vi "img test9(track 2_ num of particles).vi"() -> ()   [LabVIEW 2013]
uses:
  <vilib>/vision/NI_Vision_Development_Module.lvlib
panel:
  out "Array":i32[](array[numeric])
  in  "OK Button":bool
  out "Waveform Graph":i32[](graph)
  out "Waveform Chart":i32(graph)
  in  "frame jump":i32=3
  in  "milliseconds to wait":u32=200
  in  "start":i32
  out "Image 5":T1(plugin-control)
  out "Image 3":T1(plugin-control)
  in  "Range":cluster{"Lower value":sgl, "Upper value":sgl}={"Lower value"=30.0, "Upper value"=90.0} {"Upper value" format="%.2f"; "Lower value" format="%.2f"}
  out "Image 2":T1(plugin-control)
  in  "AVI Path":path=path "C:/Users/Kokum Weeratunga/Desktop/img processing/ChongWei vs LinDan (japan open 2010).avi"
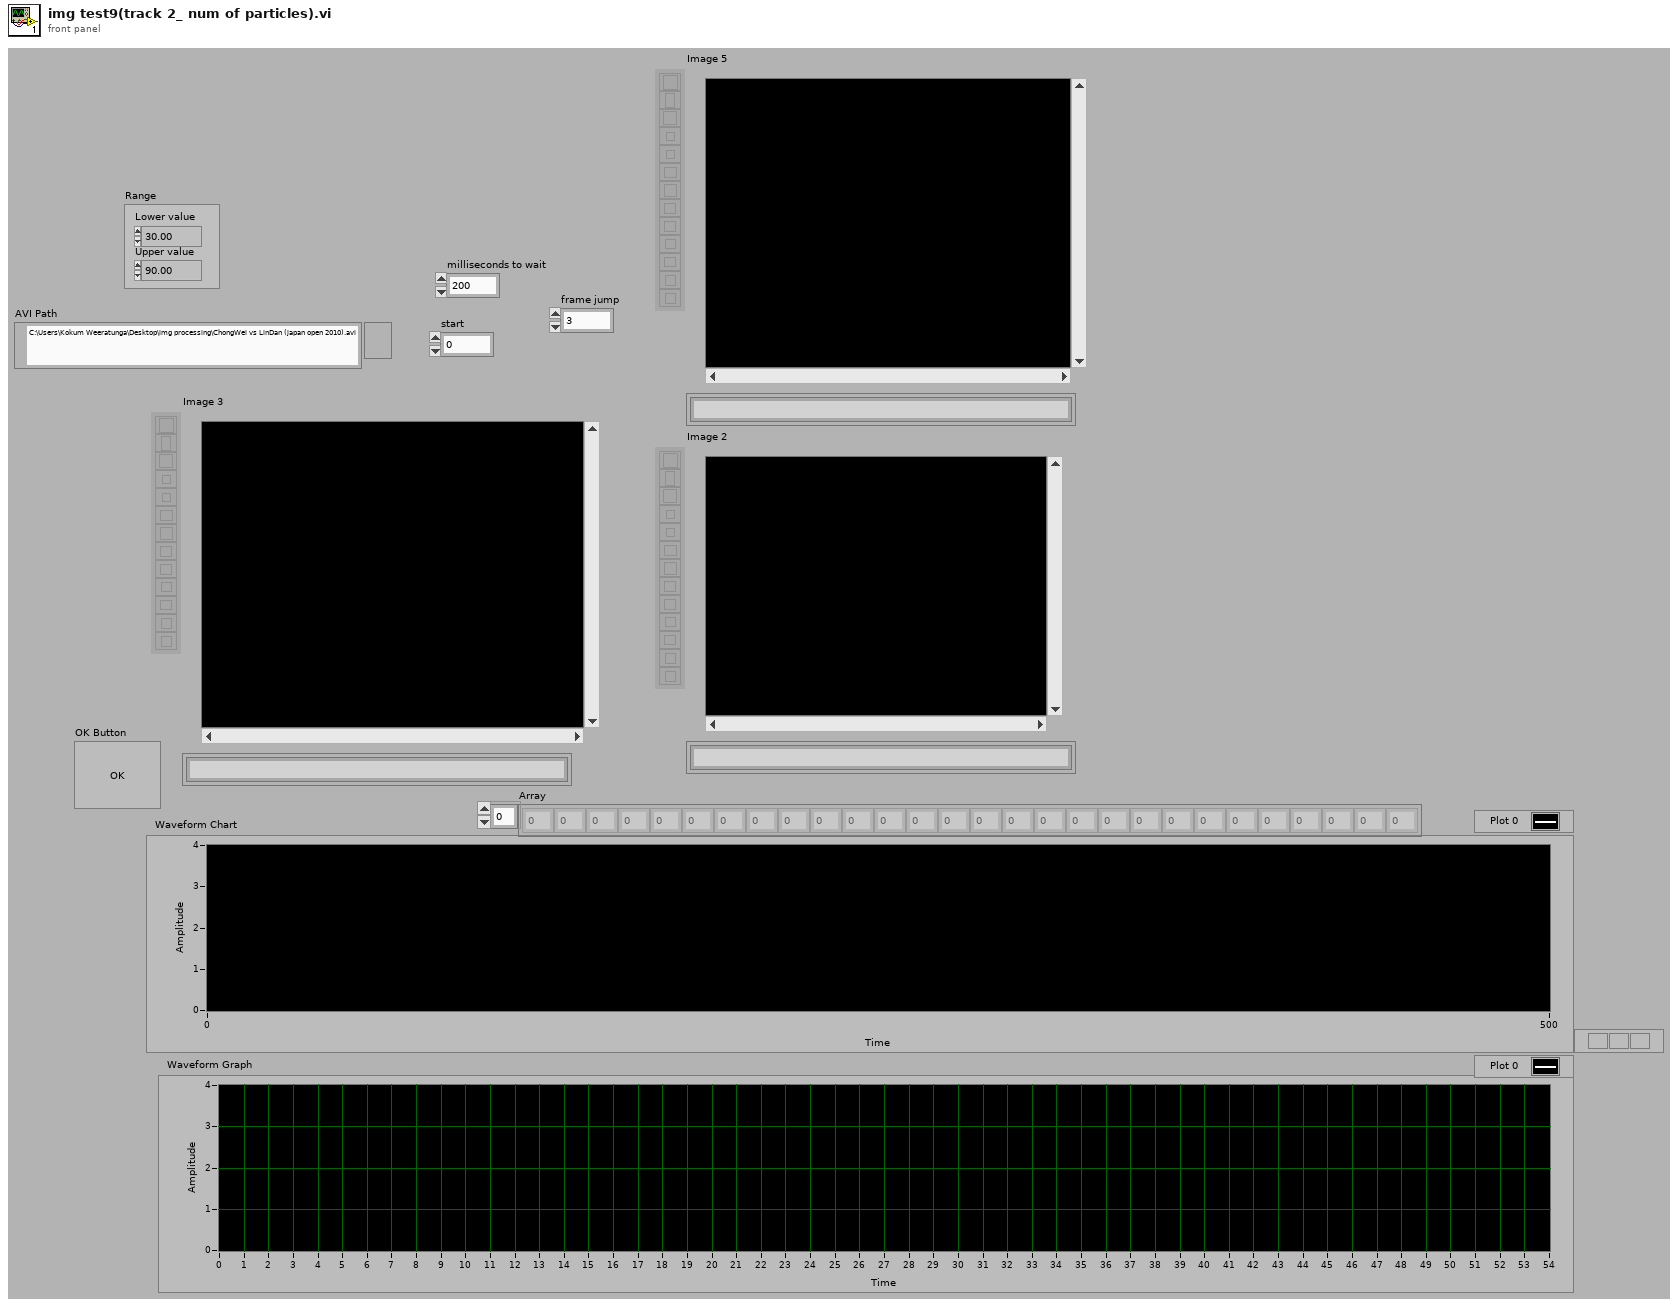
[diagram p1: front panel]
types:
  T1 = typedef "IMAQ Image.ctl" = refnum<image>
  T2 = typedef "Image Type" = u32
  T3 = typedef "AviRefnum.ctl" = refnum<k1>
  T4 = enum32{"AutoM", "Close", "Dilate", "Erode", "Gradient", "Gradient out", "Gradient in", "Hit miss", "Open", "PClose", "POpen", "Thick", "Thin"}
  T5 = enum32{"AutoM", "Close", "Dilate", "Erode", "Gradient", "Gradient in", "Gradient out", "HitMiss", "Open", "PClose", "POpen", "Thick", "Thin"}
  T6 = typedef "Particle Parameters" = i32
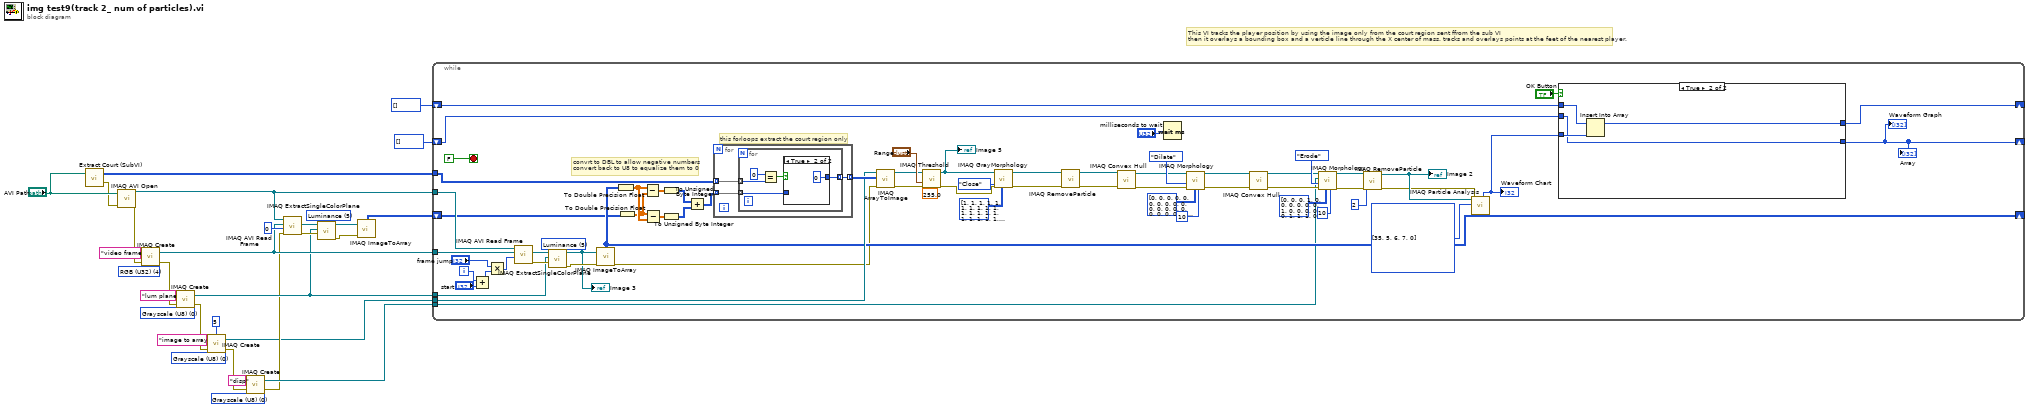
[diagram p0: block diagram]
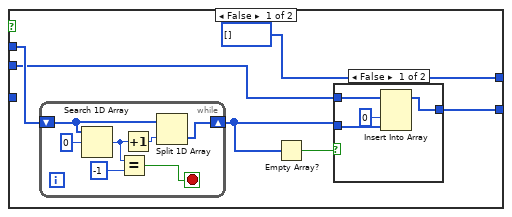
[diagram p2: hidden frame]
diagram:
  w14 = T2 0 items=["Grayscale (U8)", "Grayscale (I16)", "Grayscale (SGL)", "Complex (CSG)", "RGB (U32)", "HSL (U32)", "RGB (U64)", "Grayscale (U16)"] ("Image Type")
  w22 = 5 items=["Red", "Green", "Blue", "Hue", "Saturation", "Luminance", "Value", "Intensity"] ("Color Plane")
  w24 = T2 0 items=["Grayscale (U8)", "Grayscale (I16)", "Grayscale (SGL)", "Complex (CSG)", "RGB (U32)", "HSL (U32)", "RGB (U64)", "Grayscale (U16)"] ("Image Type")
  w28 = T2 0 items=["Grayscale (U8)", "Grayscale (I16)", "Grayscale (SGL)", "Complex (CSG)", "RGB (U32)", "HSL (U32)", "RGB (U64)", "Grayscale (U16)"] ("Image Type")
  w26 = T2 4 items=["Grayscale (U8)", "Grayscale (I16)", "Grayscale (SGL)", "Complex (CSG)", "RGB (U32)", "HSL (U32)", "RGB (U64)", "Grayscale (U16)"] ("Image Type")
  # "This VI tracks the player position by using the image only from the court region sent ffrom the sub VI\nthen it overlays a bounding box and a verticle line through the X center of mass. tracks and overlays points at the feet of the nearest player."
  n1 = call "Extract Court (SubVI).vi"("AVI Path"="AVI Path") -> ("error out"=w30:errorcluster, "Court pixels out"=w4:u8[][])  [unwired: 1 in]
  n2 = call "IMAQ AVI Open"("error in (no error)"=w30, "AVI Path"="AVI Path") -> ("error out"=w10:errorcluster, "Avi Refnum"=w20:T3)  [unwired: 8 in]
  n3 = call "IMAQ Create"("Image Name"="video frame", "Image Type"=w26, "error in (no error)"=w10) -> ("New Image"=w18:T1, "error out"=w9:errorcluster)  [unwired: 2 in]
  n4 = call "IMAQ Create"("Image Name"="lum plane", "Image Type"=w28, "error in (no error)"=w9) -> ("New Image"=w17:T1, "error out"=w8:errorcluster)  [unwired: 2 in]
  n5 = call "IMAQ Create"("Border Size"=5, "Image Name"="image to array", "Image Type"=w24, "error in (no error)"=w8) -> ("New Image"=w3:T1, "error out"=w7:errorcluster)  [unwired: 1 in]
  n6 = call "IMAQ Create"("Image Name"="disp", "Image Type"=w14, "error in (no error)"=w7) -> ("New Image"=w12:T1, "error out"=w6:errorcluster)  [unwired: 2 in]
  n7 = call "IMAQ AVI Read Frame"("error in (no error)"=w6, "Frame Number"=u32 0, "Image"=w18, "Avi Refnum"=w20) -> ("error out"=w21:errorcluster, "Image Out"=w23:T1)  [unwired: 4 in, 2 out]
  n8 = call "IMAQ ExtractSingleColorPlane"("Color Plane"=w22, "error in (no error)"=w21, "Image Dst"=w17, "Image Src"=w23) -> ("error out"=w11:errorcluster, "Image Dst Out"=w15:T1)  [unwired: 6 in]
  n9 = call "IMAQ ImageToArray"("error in (no error)"=w11, "Image"=w15) -> ("Image Pixels (U8)"=w16:u8[][])  [unwired: 2 in, 4 out]
  n10 = while {
    tunnel: w20 -> [w94]
    tunnel: w18 -> [w44]
    tunnel: w4 -> [w93]
    tunnel: w17 -> [w46]
    tunnel: w3 -> [w86]
    shift-right: [w85] -> _
    shift-left: w16 -> [w84]
    tunnel: w12 -> [w48]
    shift-right: [w40] -> _
    shift-left: i32[] [] -> [w41]
    shift-right: [w37] -> _
    shift-left: i32[] [] -> [w38]
    i -> [w77]
    stop <- FALSE stop-if-true
    w47 = T6[] [35, 5, 6, 7, 0] items=["Center of Mass X", "Center of Mass Y", "First Pixel X", "First Pixel Y", "Bounding Rect Left", "Bounding Rect Top", "Bounding Rect Right", "Bounding Rect Bottom", "Max Feret Diameter Start X", "Max Feret Diameter Start Y", "Max Feret Diameter End X", "Max Feret Diameter End Y", "Max Horiz. Segment Length Left", "Max Horiz. Segment Length Right", "Max Horiz. Segment Length Row", "-", "Bounding Rect Width", "Bounding Rect Height", "Bounding Rect Diagonal", "Perimeter", "Convex Hull Perimeter", "Holes' Perimeter", "Max Feret Diameter", "Equivalent Ellipse Major Axis", "Equivalent Ellipse Minor Axis", "Equivalent Ellipse Minor Axis (Feret)", "Equivalent Rect Long Side", "Equivalent Rect Short Side", "Equivalent Rect Diagonal", "Equivalent Rect Short Side (Feret)", "Average Horiz. Segment Length", "Average Vert. Segment Length", "Hydraulic Radius", "Waddel Disk Diameter", "-", "Area", "Holes' Area", "Particle & Holes' Area", "Convex Hull Area", "Image Area", "-", "Number of Holes", "Number of Horiz. Segments", "Number of Vert. Segments", "-", "Orientation", "Max Feret Diameter Orientation", "-", "% Area/Image Area", "% Area/(Particle & Holes' Area)", "Ratio of Equivalent Ellipse Axes", "Ratio of Equivalent Rect Sides", "-", "Elongation Factor", "Compactness Factor", "Heywood Circularity Factor", "Type Factor", "-", "Sum X", "Sum Y", "Sum XX", "Sum XY", "Sum YY", "Sum XXX", "Sum XXY", "Sum XYY", "Sum YYY", "-", "Moment of Inertia XX", "Moment of Inertia XY", "Moment of Inertia YY", "Moment of Inertia XXX", "Moment of Inertia XXY", "Moment of Inertia XYY", "Moment of Inertia YYY", "Norm. Moment of Inertia XX", "Norm. Moment of Inertia XY", "Norm. Moment of Inertia YY", "Norm. Moment of Inertia XXX", "Norm. Moment of Inertia XXY", "Norm. Moment of Inertia XYY", "Norm. Moment of Inertia YYY", "Hu Moment 1", "Hu Moment 2", "Hu Moment 3", "Hu Moment 4", "Hu Moment 5", "Hu Moment 6", "Hu Moment 7"] ("Pixel Measurements")
    w95 = 5 items=["Red", "Green", "Blue", "Hue", "Saturation", "Luminance", "Value", "Intensity"] ("Color Plane")
    # "convrt to DBL to allow negative numbers\nconvert back to U8 to equalize them to 0"
    # "this forloops extract the court region only"
    n11 = Add(x=w77, y="start") -> (x+y=w76:i32)
    n12 = Multiply(x="frame jump", y=w76) -> (x*y=w90:i32)
    n13 = call "IMAQ AVI Read Frame"("Frame Number"=w90, "Image"=w44, "Avi Refnum"=w94) -> ("error out"=w96:errorcluster, "Image Out"=w45:T1)  [unwired: 5 in, 2 out]
    n14 = call "IMAQ ExtractSingleColorPlane"("Color Plane"=w95, "error in (no error)"=w96, "Image Dst"=w46, "Image Src"=w45) -> ("error out"=w70:errorcluster, "Image Dst Out"=w43:T1)  [unwired: 6 in]
    "Image 3" <- w43
    n15 = call "IMAQ ImageToArray"("error in (no error)"=w70, "Image"=w43) -> ("error out"=w69:errorcluster, "Image Pixels (U8)"=w85:u8[][])  [unwired: 2 in, 3 out]
    n16 = To Double Precision Float(number=w85) -> (double precision float=w74:dbl[][])
    n17 = To Double Precision Float(number=w84) -> (double precision float=w73:dbl[][])
    n18 = Subtract(x=w74, y=w73) -> (x-y=w72:dbl[][])
    n19 = Subtract(x=w73, y=w74) -> (x-y=w71:dbl[][])
    n20 = To Unsigned Byte Integer(number=w72) -> (unsigned 8bit integer=w83:u8[][])
    n21 = To Unsigned Byte Integer(number=w71) -> (unsigned 8bit integer=w82:u8[][])
    n22 = Add(x=w83, y=w82) -> (x+y=w81:u8[][])
    n23 = for {
      tunnel: w93 -> [w121] mode=indexing
      tunnel: [w120] -> w91 mode=indexing
      tunnel: w81 -> [w119] mode=indexing
      n24 = for {
        tunnel: w121 -> [w126] mode=indexing
        tunnel: [w123] -> w120 mode=indexing
        tunnel: w119 -> [w122] mode=indexing
        n25 = Equal?(x=u8 0, y=w126) -> (x = y?=w124:bool)
        n26 = case shown="True" w124 {
          tunnel: [w127 u8 0 ("x")] -> w123
          tunnel: w122 -> [w127 _]
          frame False {
          }
          frame True {
          }
        }
      }
    }
    n27 = call "IMAQ ArrayToImage"("error in (no error)"=w69, "Image Pixels (U8)"=w91, "Image"=w86) -> ("error out"=w68:errorcluster, "Image Out"=w50:T1)  [unwired: 7 in]
    n28 = call "IMAQ Threshold"("Replace Value"=sgl 255.0, "error in (no error)"=w68, "Range"="Range", "Image Src"=w50) -> ("error out"=w67:errorcluster, "Image Dst Out"=w80:T1)  [unwired: 6 in]
    "Image 5" <- w80
    n29 = call "IMAQ GrayMorphology"("Structuring Element"=i32[][] [[1, 1, 1, 1, 1, 1, 1, 1, 1], [1, 1, 1, 1, 1, 1, 1, 1, 1], [1, 1, 1, 1, 1, 1, 1, 1, 1], [1, 1, 1, 1, 1, 1, 1, 1, 1], [1, 1, 1, 1, 1, 1, 1, 1, 1], [1, 1, 1, 1, 1, 1, 1, 1, 1], [1, 1, 1, 1, 1, 1, 1, 1, 1], [1, 1, 1, 1, 1, 1, 1, 1, 1], [1, 1, 1, 1, 1, 1, 1, 1, 1]], "error in (no error)"=w67, "Operation"=T5."Close", "Image Src"=w80) -> ("error out"=w65:errorcluster, "Image Dst Out"=w66:T1)  [unwired: 6 in]
    n30 = call "IMAQ RemoveParticle"("error in (no error)"=w65, "Image Src"=w66) -> ("error out"=w64:errorcluster, "Image Dst Out"=w63:T1)  [unwired: 8 in]
    n31 = call "IMAQ Convex Hull"("error in (no error)"=w64, "Image Src"=w63) -> ("error out"=w59:errorcluster, "Image Dst Out"=w49:T1)  [unwired: 8 in]
    n32 = Wait (ms)(milliseconds to wait="milliseconds to wait") -> ()  [unwired: 1 out]
    n33 = call "IMAQ Morphology"("Number of iterations (1)"=10, "Structuring Element"=i32[][] [[0, 0, 0, 0, 0, 0, 0], [0, 0, 0, 0, 0, 0, 0], [0, 0, 0, 0, 0, 0, 0], [0, 0, 0, 0, 0, 0, 0], [0, 0, 1, 1, 1, 0, 0], [0, 0, 0, 1, 0, 0, 0], [0, 0, 0, 1, 0, 0, 0]], "error in (no error)"=w59, "Operation"=T4."Dilate", "Image Src"=w49) -> ("error out"=w53:errorcluster, "Image Dst Out"=w54:T1)  [unwired: 5 in]
    n34 = call "IMAQ Convex Hull"("error in (no error)"=w53, "Image Src"=w54) -> ("error out"=w51:errorcluster, "Image Dst Out"=w52:T1)  [unwired: 8 in]
    n35 = call "IMAQ Morphology"("Number of iterations (1)"=10, "Structuring Element"=i32[][] [[0, 0, 0, 1, 0, 0, 0], [0, 0, 0, 1, 0, 0, 0], [0, 0, 1, 1, 1, 0, 0], [0, 0, 0, 0, 0, 0, 0], [0, 0, 0, 0, 0, 0, 0], [0, 0, 0, 0, 0, 0, 0], [0, 0, 0, 0, 0, 0, 0]], "error in (no error)"=w51, "Operation"=T4."Erode", "Image Dst"=w48, "Image Src"=w52) -> ("error out"=w34:errorcluster, "Image Dst Out"=w36:T1)  [unwired: 4 in]
    n36 = call "IMAQ RemoveParticle"("error in (no error)"=w34, "Number of Erosion"=2, "Image Src"=w36) -> ("error out"=w33:errorcluster, "Image Dst Out"=w35:T1)  [unwired: 7 in]
    "Image 2" <- w35
    n37 = call "IMAQ Particle Analysis"("error in (no error)"=w33, "Pixel Measurements"=w47, "Image"=w35) -> ("Number of Particles"=w42:i32)  [unwired: 3 in, 5 out]
    "Waveform Chart" <- w42
    n38 = case shown="True" "OK Button" {
      tunnel: w42 -> [_ w118]
      tunnel: w41 -> [w101 w117]
      tunnel: [i32[] [] w116] -> w40
      tunnel: [w100 w115] -> w37
      tunnel: w38 -> [w99 w115]
      frame False {
        n39 = while {
          shift-right: [w112] -> w98
          shift-left: w101 -> [w113]
          stop <- w110 stop-if-true
          n40 = Search 1D Array(1D array=w113, element=0) -> (index of element=w108:i32)  [unwired: 1 in]
          n41 = Equal?(x=w108, y=-1) -> (x = y?=w110:bool)
          n42 = Increment(x=w108) -> (x+1=w109:i32)
          n43 = Split 1D Array(array=w113, index=w109) -> (second subarray=w112:i32[])  [unwired: 1 out]
        }
        n44 = Empty Array?(array=w98) -> (empty?=w97:bool)
        n45 = case shown="False" w97 {
          tunnel: [w106 w107] -> w100
          tunnel: w99 -> [w105 w107]
          tunnel: w98 -> [w104 _]
          frame False {
            n46 = Insert Into Array(array=w105, new element #1=0 ("new element/subarray"), new element #2=w104) -> (w106:i32[])  [unwired: 1 in]
          }
          frame True {
          }
        }
      }
      frame True {
        n47 = Insert Into Array(array=w117, new element=w118) -> (w116:i32[])  [unwired: 1 in]
      }
    }
    "Waveform Graph" <- w37
    "Array" <- w37
  }
